vi "Read Shifters from File.vi"(8 "error in (no error)":errorcluster, 10 "XML File Path":path, 11 "Shifters in":refnum<class "Shifters.lvclass">) -> (0 "error out":errorcluster, 3 "Shifters out":refnum<class "Shifters.lvclass">)   [LabVIEW 2013]
uses:
  Shifters.lvclass
  <vilib>/Utility/xml.llb/Read From XML File(string).vi
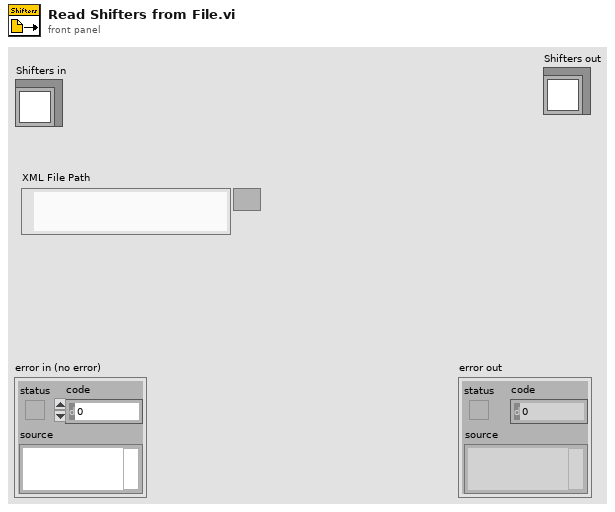
[diagram p1: front panel]
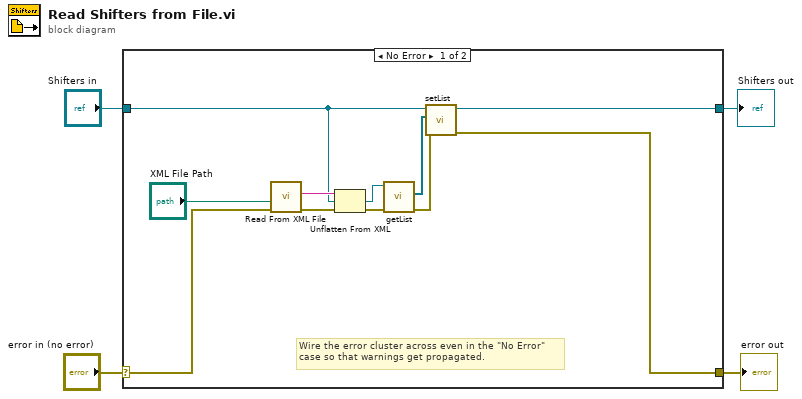
[diagram p0: block diagram]
diagram:
  n1 = case shown="No Error" "error in (no error)" {
    selector: "error in (no error)" -> [w14 w17]
    tunnel: [w7 w17] -> w3
    tunnel: [w8 w16] -> w1
    tunnel: "Shifters in" -> [w5 w16]
    frame No Error {
      # "Wire the error cluster across even in the \"No Error\"\ncase so that warnings get propagated."
      n2 = call-poly <vilib>:"Read From XML File.vi"("error in (no error)"=w14, "XML File Path"="XML File Path") -> ("error out"=w13:errorcluster, "XML Elements"=w12:string)  [unwired: 7 in, 1 out]
      n3 = Unflatten From XML(xml string=w12, type=w5, error in (no error)=w13) -> (value=w10:refnum<class "Shifters.lvclass">, error out=w11:errorcluster)
      n4 = call-dynamic "getList.vi"("error in (no error)"=w11, "Shifters in"=w10) -> ("error out"=w9:errorcluster, "list"=w6:refnum<class "Shifter.lvclass">[])  [unwired: 7 in, 1 out]
      n5 = call-dynamic "setList.vi"("error in (no error)"=w9, "list"=w6, "Shifters in"=w5) -> ("error out"=w7:errorcluster, "Shifters out"=w8:refnum<class "Shifters.lvclass">)  [unwired: 7 in]
    }
    frame Error {
    }
  }
  "error out" <- w3
  "Shifters out" <- w1
